vi "__Cloud List DoubleClick Handler.vi"(8 "error in (no error)":errorcluster, 10 "Clicked Row":i32, 11 "FileManager Data in":T1) -> (0 "error out":errorcluster, 3 "FileManager Data out":T1)   [LabVIEW 2011]
doc: "Handles the double-click operation on the Cloud List."
uses:
  __File manager Data type.ctl
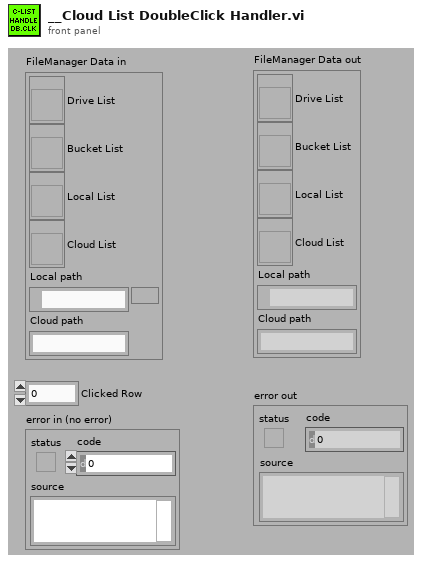
[diagram p1: front panel]
types:
  T1 = typedef "__File manager Data type.ctl" = cluster{"Drive List":refnum<vi>, "Bucket List":refnum<vi>, "Local List":refnum<vi>, "Cloud List":refnum<vi>, "Local path":path, "Cloud path":string}
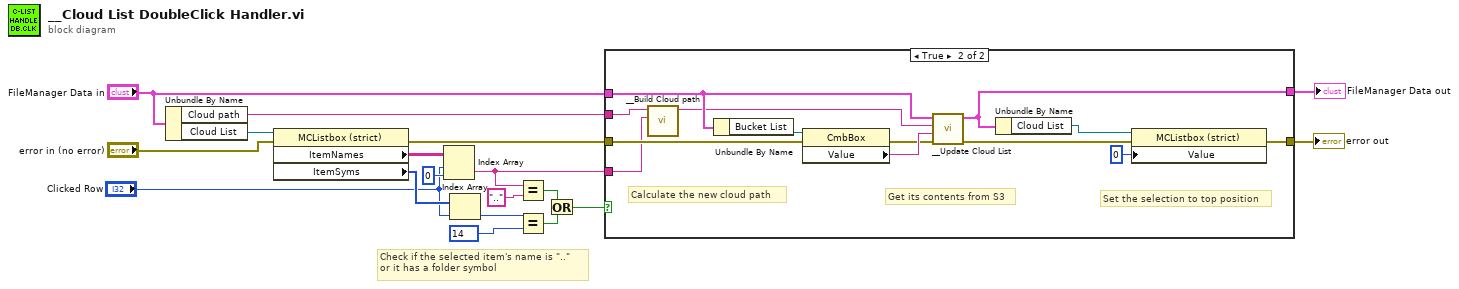
[diagram p0: block diagram]
diagram:
  # "Check if the selected item's name is \"..\"\nor it has a folder symbol"
  n1 = Unbundle By Name("FileManager Data in") -> ("Cloud path"=w6:string, "Cloud List"=w11:refnum<vi>)
  n2 = property class="MCListbox (strict)"(reference=w11, error in="error in (no error)") -> (error out=w16:errorcluster, "ItemNames"=w18:string[][], "ItemSyms"=w10:i32[])  [unwired: 1 out]
  n3 = Index Array(array=w18, index (row)="Clicked Row", index (col)=0 ("disabled index (col)")) -> (element=w5:string)
  n4 = Index Array(array=w10, index="Clicked Row") -> (element=w8:i32)
  n5 = Equal?(x=w5, y="..") -> (x = y?=w3:bool)
  n6 = Equal?(x=w8, y=14) -> (x = y?=w2:bool)
  n7 = Or(x=w3, y=w2) -> (x .or. y?=w1:bool)
  n8 = case shown="True" w1 {
    tunnel: w16 -> [w20 w24]
    tunnel: "FileManager Data in" -> [w19 w28]
    tunnel: [w19 w30] -> w14
    tunnel: [w20 w31] -> w13
    tunnel: w6 -> [_ w23]
    tunnel: w5 -> [_ w22]
    frame False {
      # "This is not a folder, so double-click won't have any effects."
    }
    frame True {
      # "Set the selection to top position"
      # "Get its contents from S3"
      # "Calculate the new cloud path"
      n9 = call "__Build Cloud path.vi"("New Path element"=w22, "Current Cloud path"=w23) -> ("New Cloud path"=w21:string)  [unwired: 9 in]
      n10 = Unbundle By Name(w28) -> ("Bucket List"=w27:refnum<vi>)
      n11 = property class="CmbBox"(reference=w27, error in=w24) -> (error out=w25:errorcluster, "Value"=w26:string)  [unwired: 1 out]
      n12 = call "__Update Cloud List.vi"("error in (no error)"=w25, "Bucket"=w26, "Path to list"=w21, "FileManager Ctl Refs in"=w28) -> ("error out"=w33:errorcluster, "FileManager Ctl Refs out"=w30:T1)  [unwired: 6 in]
      n13 = Unbundle By Name(w30) -> ("Cloud List"=w29:refnum<vi>)
      n14 = property class="MCListbox (strict)"(reference=w29, error in=w33, "Value"=0) -> (error out=w31:errorcluster)  [unwired: 1 out]
    }
  }
  "FileManager Data out" <- w14
  "error out" <- w13
